vi "BMP180 Init.vi"(7 "I2C Channel":u8, 8 "error in (no error)":errorcluster, 9 "BMP180 Config Options":T1={"I2C"={"Slave Address"=64, "Channel"=0}, "Mode"=enum."Ultra Low Power", "Cal Coefs"={"AC1"={"Addr:"=170, "Val:"=0}, "AC2"={"Addr:"=172, "Val:"=0}, "AC3"={"Addr:"=174, "Val:"=0}, "AC4"={"Addr:"=176, "Val:"=0}, "AC5"={"Addr:"=178, "Val:"=0}, "AC6"={"Addr:"=180, "Val:"=0}, "B1"={"Addr:"=182, "Val:"=0}, "B2"={"Addr:"=184, "Val:"=0}, "MB"={"Addr:"=186, "Val:"=0}, "MC"={"Addr:"=188, "Val:"=0}, "MD"={"Addr:"=190, "Val:"=0}}, "Online"=FALSE} {"I2C"."Slave Address" format="%.0x"; "Cal Coefs"."MD"."Val:" format="%04x"; "Cal Coefs"."MD"."Addr:" format="%02x"; "Cal Coefs"."MC"."Val:" format="%04x"; "Cal Coefs"."MC"."Addr:" format="%02x"; "Cal Coefs"."MB"."Val:" format="%04x"; "Cal Coefs"."MB"."Addr:" format="%02x"; "Cal Coefs"."B2"."Val:" format="%04x"; "Cal Coefs"."B2"."Addr:" format="%02x"; "Cal Coefs"."B1"."Val:" format="%04x"; "Cal Coefs"."B1"."Addr:" format="%02x"; "Cal Coefs"."AC6"."Val:" format="%04x"; "Cal Coefs"."AC6"."Addr:" format="%02x"; "Cal Coefs"."AC5"."Val:" format="%04x"; "Cal Coefs"."AC5"."Addr:" format="%02x"; "Cal Coefs"."AC4"."Val:" format="%04x"; "Cal Coefs"."AC4"."Addr:" format="%02x"; "Cal Coefs"."AC3"."Val:" format="%04x"; "Cal Coefs"."AC3"."Addr:" format="%02x"; "Cal Coefs"."AC2"."Val:" format="%04x"; "Cal Coefs"."AC2"."Addr:" format="%02x"; "Cal Coefs"."AC1"."Val:" format="%04x"; "Cal Coefs"."AC1"."Addr:" format="%02x"}, 10 "I2C Slave Address":u8=119 format="%.0x", 11 "LINX Resource in":T2) -> (0 "error out":errorcluster, 1 "BMP180 Config Options":T1={"I2C"={"Slave Address"=64, "Channel"=0}, "Mode"=enum."Ultra Low Power", "Cal Coefs"={"AC1"={"Addr:"=0, "Val:"=0}, "AC2"={"Addr:"=0, "Val:"=0}, "AC3"={"Addr:"=0, "Val:"=0}, "AC4"={"Addr:"=0, "Val:"=0}, "AC5"={"Addr:"=0, "Val:"=0}, "AC6"={"Addr:"=0, "Val:"=0}, "B1"={"Addr:"=0, "Val:"=0}, "B2"={"Addr:"=0, "Val:"=0}, "MB"={"Addr:"=0, "Val:"=0}, "MC"={"Addr:"=0, "Val:"=0}, "MD"={"Addr:"=0, "Val:"=0}}, "Online"=FALSE} {"I2C"."Slave Address" format="%.0x"; "Cal Coefs"."MD"."Val:" format="%04x"; "Cal Coefs"."MD"."Addr:" format="%02x"; "Cal Coefs"."MC"."Val:" format="%04x"; "Cal Coefs"."MC"."Addr:" format="%02x"; "Cal Coefs"."MB"."Val:" format="%04x"; "Cal Coefs"."MB"."Addr:" format="%02x"; "Cal Coefs"."B2"."Val:" format="%04x"; "Cal Coefs"."B2"."Addr:" format="%02x"; "Cal Coefs"."B1"."Val:" format="%04x"; "Cal Coefs"."B1"."Addr:" format="%02x"; "Cal Coefs"."AC6"."Val:" format="%04x"; "Cal Coefs"."AC6"."Addr:" format="%02x"; "Cal Coefs"."AC5"."Val:" format="%04x"; "Cal Coefs"."AC5"."Addr:" format="%02x"; "Cal Coefs"."AC4"."Val:" format="%04x"; "Cal Coefs"."AC4"."Addr:" format="%02x"; "Cal Coefs"."AC3"."Val:" format="%04x"; "Cal Coefs"."AC3"."Addr:" format="%02x"; "Cal Coefs"."AC2"."Val:" format="%04x"; "Cal Coefs"."AC2"."Addr:" format="%02x"; "Cal Coefs"."AC1"."Val:" format="%04x"; "Cal Coefs"."AC1"."Addr:" format="%02x"}, 3 "LINX Resource out":T2)   [LabVIEW 2017]
uses:
  <vilib>/MakerHub/LINX/Private/Type Defs/LINX Ref.ctl
  <vilib>/MakerHub/LINX/Private/Type Defs/Platform.ctl
  <vilib>/MakerHub/LINX/Private/Type Defs/Interface.ctl
  <vilib>/MakerHub/LINX/Private/Device/Type Defs/LINX Device Config.ctl
  <vilib>/MakerHub/LINX/Private/Device/Type Defs/TCP Config.ctl
  <vilib>/MakerHub/LINX/Private/Device/Type Defs/Channels.ctl
  BMP180 Config Options.ctl
  <vilib>/MakerHub/LINX/LMH-LINX.lvlib
  <vilib>/MakerHub/LINX/Private/Device/Device.lvlib
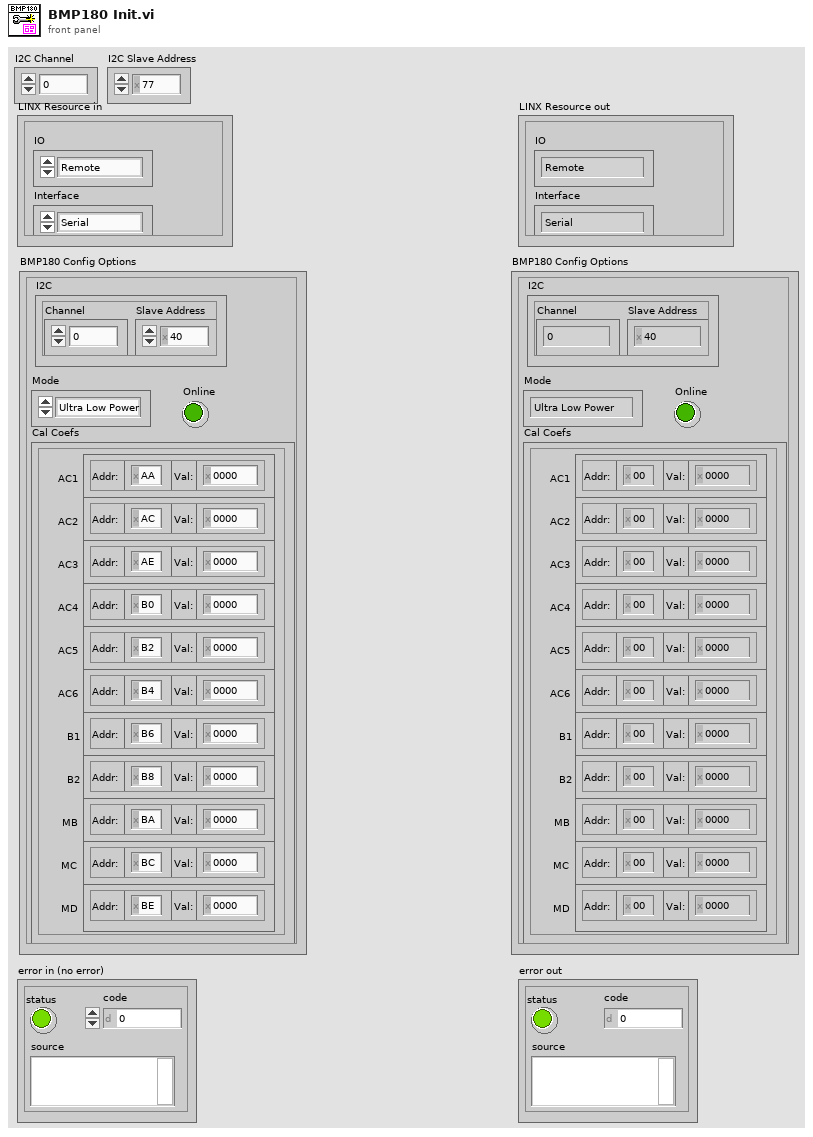
[diagram p1: front panel]
types:
  T1 = typedef "BMP180 Config Options.ctl" = cluster{"I2C":cluster{"Slave Address":u8, "Channel":u8}, "Mode":enum8{"Ultra Low Power", "Standard", "High Resolution", "Ultra High Resolution"}, "Cal Coefs":cluster{"AC1":cluster{"Addr:":u8, "Val:":u16}, "AC2":cluster{"Addr:":u8, "Val:":u16}, "AC3":cluster{"Addr:":u8, "Val:":u16}, "AC4":cluster{"Addr:":u8, "Val:":u16}, "AC5":cluster{"Addr:":u8, "Val:":u16}, "AC6":cluster{"Addr:":u8, "Val:":u16}, "B1":cluster{"Addr:":u8, "Val:":u16}, "B2":cluster{"Addr:":u8, "Val:":u16}, "MB":cluster{"Addr:":u8, "Val:":u16}, "MC":cluster{"Addr:":u8, "Val:":u16}, "MD":cluster{"Addr:":u8, "Val:":u16}}, "Online":bool}
  T2 = typedef "LMH-LINX.lvlib/LINX Ref.ctl" = cluster{"IO":T3, "Interface":T4, "LINX Device Config":T5}
  T3 = typedef "LMH-LINX.lvlib/Platform.ctl" = enum16{"Remote", "Local"}
  T4 = typedef "LMH-LINX.lvlib/Interface.ctl" = enum16{"Serial", "TCP"}
  T5 = typedef "LMH-LINX.lvlib/Device.lvlib/LINX Device Config.ctl" = cluster{"Interface":T4, "COM Port":refnum<visa-resource-name>, "TCP Configuration":T6, "Device Family":u8, "Device ID":u8, "Device Name":string, "TCP Ref":refnum<k5>, "Channels":T7}
  T6 = typedef "LMH-LINX.lvlib/Device.lvlib/TCP Config.ctl" = cluster{"IP Address":string, "Port":u16}
  T7 = typedef "LMH-LINX.lvlib/Channels.ctl" = cluster{"DI":u8[], "DO":u8[], "AI":u8[], "AO":u8[], "PWM":u8[], "QE":u8[], "UART":u8[], "I2C 2":u8[], "SPI":u8[], "CAN":u8[], "Servo":u8[], "AI Ref (V)":dbl, "AI Resolution (Bits)":u8, "AO Ref (V)":dbl, "AO Resolution (Bits)":u8}
  T8 = cluster{"AC1":cluster{"Addr:":u8, "Val:":u16}, "AC2":cluster{"Addr:":u8, "Val:":u16}, "AC3":cluster{"Addr:":u8, "Val:":u16}, "AC4":cluster{"Addr:":u8, "Val:":u16}, "AC5":cluster{"Addr:":u8, "Val:":u16}, "AC6":cluster{"Addr:":u8, "Val:":u16}, "B1":cluster{"Addr:":u8, "Val:":u16}, "B2":cluster{"Addr:":u8, "Val:":u16}, "MB":cluster{"Addr:":u8, "Val:":u16}, "MC":cluster{"Addr:":u8, "Val:":u16}, "MD":cluster{"Addr:":u8, "Val:":u16}}
  T9 = cluster{"[0]":cluster{"Addr:":u8, "Val:":u16}, "[1]":cluster{"Addr:":u8, "Val:":u16}, "[2]":cluster{"Addr:":u8, "Val:":u16}, "[3]":cluster{"Addr:":u8, "Val:":u16}, "[4]":cluster{"Addr:":u8, "Val:":u16}, "[5]":cluster{"Addr:":u8, "Val:":u16}, "[6]":cluster{"Addr:":u8, "Val:":u16}, "[7]":cluster{"Addr:":u8, "Val:":u16}, "[8]":cluster{"Addr:":u8, "Val:":u16}, "[9]":cluster{"Addr:":u8, "Val:":u16}, "[10]":cluster{"Addr:":u8, "Val:":u16}}
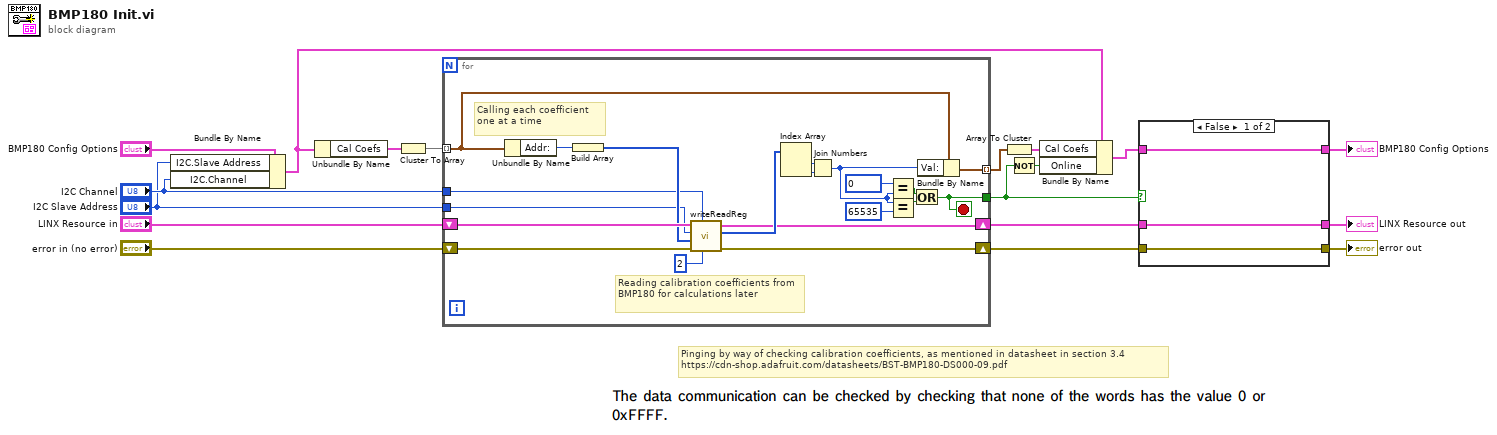
[diagram p0: block diagram]
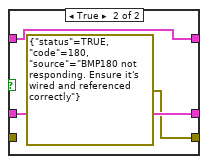
[diagram p2: hidden frame]
diagram:
  # "Pinging by way of checking calibration coefficients, as mentioned in datasheet in section 3.4\nhttps://cdn-shop.adafruit.com/datasheets/BST-BMP180-DS000-09.pdf"
  n1 = Bundle By Name(cluster="BMP180 Config Options", "I2C.Slave Address"="I2C Slave Address", "I2C.Channel"="I2C Channel") -> (w3:T1)
  n2 = Unbundle By Name(w3) -> ("Cal Coefs"=w11:T8)
  n3 = Cluster To Array(cluster=w11) -> (array=w10:cluster{"Addr:":u8, "Val:":u16}[])
  n4 = for {
    tunnel: "I2C Slave Address" -> [w23]
    tunnel: "I2C Channel" -> [w24]
    shift-right: [w20] -> w15
    shift-left: "LINX Resource in" -> [w36]
    shift-right: [w19] -> w14
    shift-left: "error in (no error)" -> [w28]
    tunnel: [w31] -> w2
    tunnel: w10 -> [w27] mode=indexing
    tunnel: [w25] -> w9 mode=indexing
    stop <- w31 stop-if-true
    # "Calling each coefficient one at a time"
    # "Reading calibration coefficients from BMP180 for calculations later"
    n5 = Unbundle By Name(w27) -> ("Addr:"=w30:u8)
    n6 = Build Array(w30) -> (w29:u8[])
    n7 = call "writeReadReg.vi"("Bytes To Read"=u8 2, "I2C Channel"=w24, "error in"=w28, "Data"=w29, "I2C Slave Address"=w23, "LINX Resource in"=w36) -> ("error out"=w19:errorcluster, "Bytes Read"=w21:u8[], "LINX Resource out"=w20:T2)  [unwired: 3 in]
    n8 = Index Array(array=w21) -> (element #1=w38:u8, element #2=w37:u8)  [unwired: 2 in]
    n9 = Join Numbers(hi=w38, lo=w37) -> ((hi.lo)=w26:u16)
    n10 = Equal?(x=u16 0 ("(hi.lo)"), y=w26) -> (x = y?=w32:bool)
    n11 = Equal?(x=w26, y=u16 65535 ("(hi.lo)")) -> (x = y?=w33:bool)
    n12 = Or(x=w32, y=w33) -> (x .or. y?=w31:bool)
    n13 = Bundle By Name(cluster=w27, "Val:"=w26) -> (w25:cluster{"Addr:":u8, "Val:":u16})
  }
  n14 = Array To Cluster(array=w9) -> (cluster=w8:T9)
  n15 = Not(x=w2) -> (.not. x?=w1:bool)
  n16 = Bundle By Name(cluster=w3, "Cal Coefs"=w8, "Online"=w1) -> (w7:T1)
  n17 = case shown="False" w2 {
    tunnel: w15 -> [w40 w44]
    tunnel: [w40 w44] -> w17
    tunnel: w14 -> [w41 _]
    tunnel: [w41 errorcluster {"status"=TRUE, "code"=180, "source"="BMP180 not responding. Ensure it's wired and referenced correctly"} ("error constant")] -> w16
    tunnel: [w39 w42] -> w13
    tunnel: w7 -> [w39 w42]
    frame False {
    }
    frame True {
    }
  }
  "error out" <- w16
  "LINX Resource out" <- w17
  "BMP180 Config Options" <- w13
